vi "Monitors_EPR_v02.vi"(0 "IIR filter specifications":T1={"Topology"=enum."Butterworth", "Type"=enum."Lowpass", "Order"=1, "Lower Fc"=100.0, "Upper Fc"=200.0, "PB Ripple"=1.0, "SB Attenuation"=60.0} {"PB Ripple" format="%0.2f"; "SB Attenuation" format="%0.2f"; "Lower Fc" format="%0.2p"; "Upper Fc" format="%0.2p"}, 3 "Wait(mSec)":u32 caption="Count(mSec)", 5 "reset SN":bool, 7 "mode 2 polarity(T=+ve)":bool, 9 "Shot noise start":bool, 11 "wfm":waveform(dbl)[](array[waveform]), 12 "mode 3 polarity(T=+ve)":bool) -> (4 "Var(x1-x2/sqrt(2)-x3/sqrt(2))":dbl, 6 "Var(x2-x1/sqrt(2)-x3/sqrt(2))":dbl, 8 "Var(x3-x1/sqrt(2)-x2/sqrt(2))":dbl)   [LabVIEW 2013]
uses:
  <vilib>/Analysis/5stat.llb/RMS (DBL).vi
  shotnoise.vi
  <vilib>/measure/maspectr.llb/FFT Spectrum (Mag-Phase) for N Chan.vi
  <vilib>/measure/matone.llb/Extract Single Tone Information N Chan.vi
  <vilib>/measure/macond.llb/IIR Filter for N Chan.vi
  <vilib>/measure/NI_MAPro.lvlib
  <vilib>/Analysis/NI_AALPro.lvlib
panel:
  out "Waveform Graph 2":cluster{"f0":dbl, "df":dbl, "magnitude":dbl[]}[](graph)
  out "detected frequencies":dbl[](array[numeric]) format="%.2p"
  out "ch12":dbl
  out "ch02":dbl
  out "ch01":dbl
  out "Waveform Graph":waveform(dbl)[](graph)
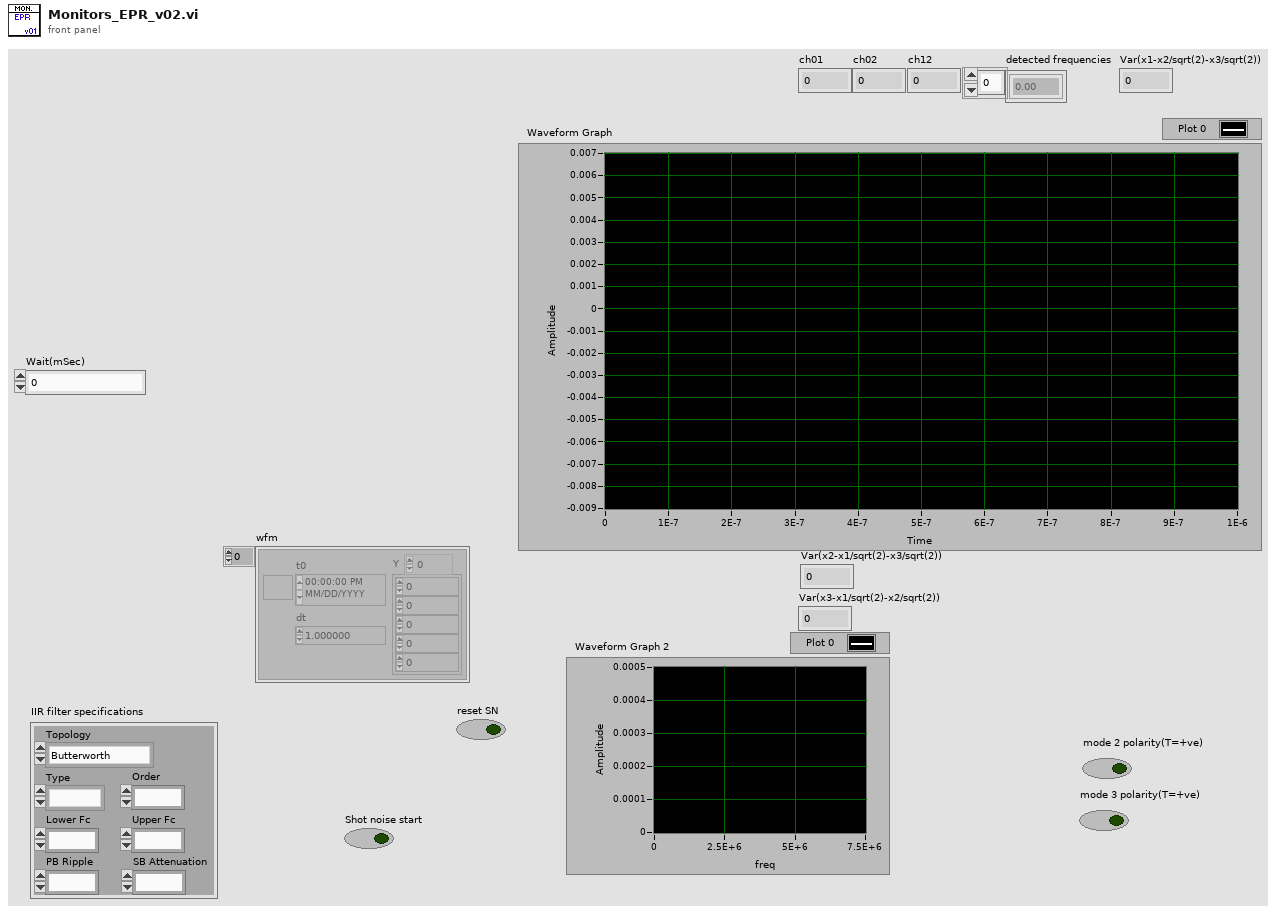
[diagram p1: front panel]
types:
  T1 = cluster{"Topology":enum16{"Off", "Butterworth", "Chebyshev", "Inverse Chebyshev", "Elliptic", "Bessel"}, "Type":enum16{"Lowpass", "Highpass", "Bandpass", "Bandstop"}, "Order":i32, "Lower Fc":dbl, "Upper Fc":dbl, "PB Ripple":dbl, "SB Attenuation":dbl}
  T2 = cluster{"approx freq. (optional)":dbl, "search (+/- % of Fsampl.)":dbl}
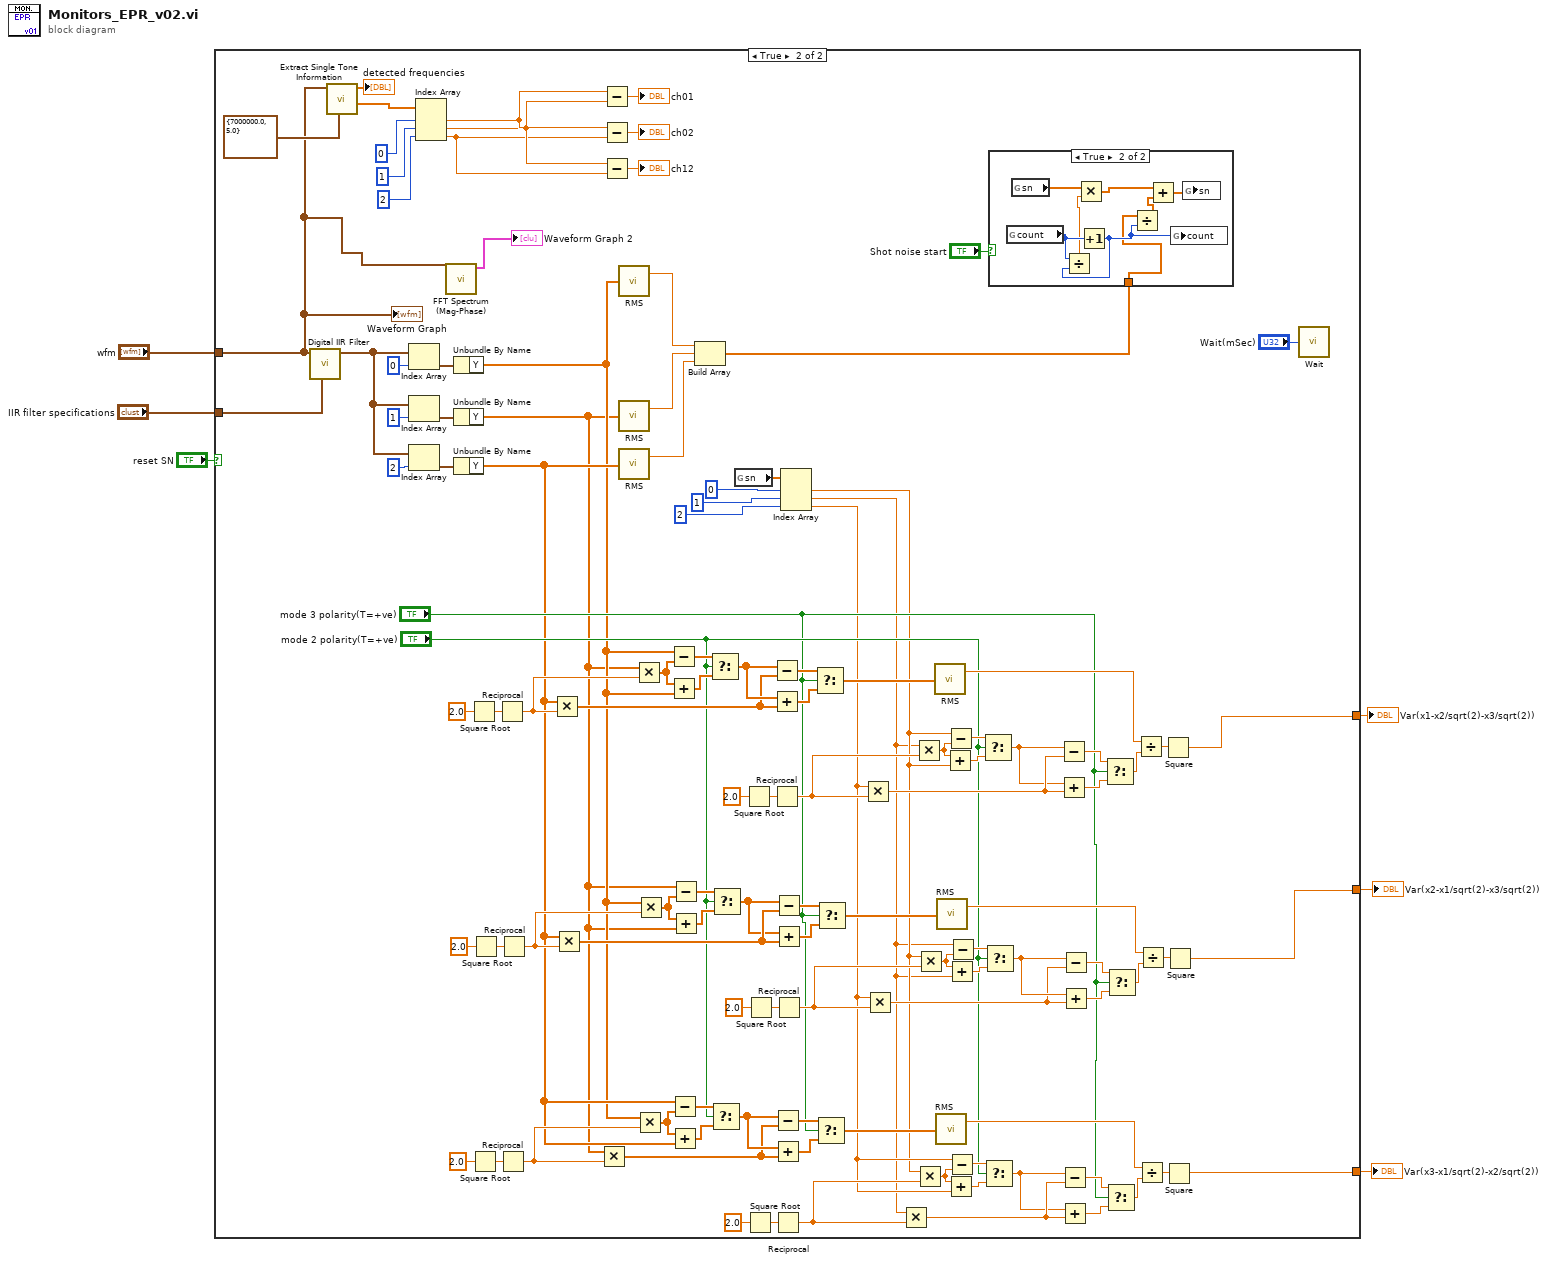
[diagram p0: block diagram]
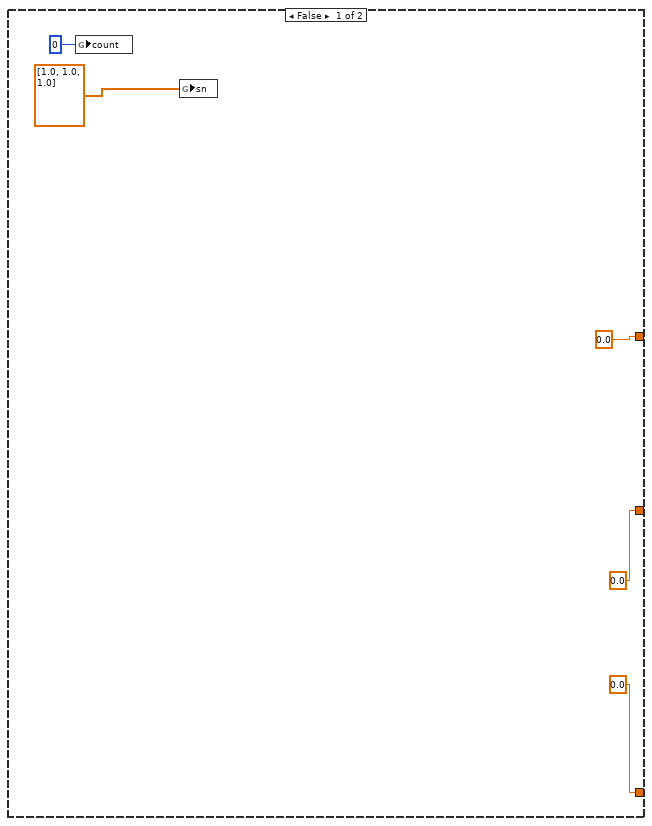
[diagram p2: hidden frame]
diagram:
  n1 = case shown="True" "reset SN" {
    tunnel: "IIR filter specifications" -> [_ w126]
    tunnel: "wfm" -> [_ w95]
    tunnel: [0.0 w89] -> w3
    tunnel: [0.0 w45] -> w2
    tunnel: [0.0 w12] -> w1
    frame False {
      n2 = global write "shotnoise.vi" "count"(i64 0 ("count")) -> ()
      n3 = global write "shotnoise.vi" "sn"(dbl[] [1.0, 1.0, 1.0] ("sn")) -> ()
    }
    frame True {
      n4 = call-poly <vilib>:"Digital IIR Filter.vi"("IIR filter specifications"=w126, "signal(s) in"=w95) -> ("signal(s) out"=w114:waveform(dbl)[])  [unwired: 4 in, 5 out]
      n5 = call-poly <vilib>:"Extract Single Tone Information.vi"("advanced search"=T2 {"approx freq. (optional)"=7000000.0, "search (+/- % of Fsampl.)"=5.0}, "time signals in"=w95) -> ("detected phases (deg)"=w105:dbl[], "detected frequencies"=→"detected frequencies":dbl[])  [unwired: 4 in, 4 out]
      n6 = Index Array(array=w114, index=0) -> (element=w118:waveform(dbl))
      n7 = Index Array(array=w114, index=1) -> (element=w121:waveform(dbl))
      n8 = Index Array(array=w114, index=2) -> (element=w113:waveform(dbl))
      n9 = Index Array(array=w105, index #1=0 ("index"), index #2=1 ("index"), index #3=2 ("index")) -> (element #1=w104:dbl, element #2=w103:dbl, element #3=w102:dbl)
      n10 = call-poly <vilib>:"FFT Spectrum (Mag-Phase).vi"("time signals"=w95) -> ("magnitudes"=→"Waveform Graph 2":cluster{"f0":dbl, "df":dbl, "magnitude":dbl[]}[])  [unwired: 6 in, 4 out]
      n11 = Unbundle By Name(w118) -> ("Y"=w16:dbl[])
      n12 = Unbundle By Name(w121) -> ("Y"=w13:dbl[])
      n13 = Unbundle By Name(w113) -> ("Y"=w18:dbl[])
      n14 = Square Root(x=2.0) -> (sqrt(x)=w93:dbl)
      n15 = Square Root(x=2.0) -> (sqrt(x)=w43:dbl)
      n16 = Square Root(x=2.0) -> (sqrt(x)=w47:dbl)
      n17 = Reciprocal(x=w93) -> (1/x=w87:dbl)
      n18 = Reciprocal(x=w43) -> (1/x=w38:dbl)
      n19 = Reciprocal(x=w47) -> (1/x=w52:dbl)
      n20 = Multiply(x=w18, y=w87) -> (x*y=w81:dbl[])
      n21 = Multiply(x=w18, y=w52) -> (x*y=w58:dbl[])
      n22 = Multiply(x=w13, y=w38) -> (x*y=w32:dbl[])
      n23 = Subtract(x=w104, y=w103) -> (x-y=→"ch01":dbl)
      n24 = Subtract(x=w104, y=w102) -> (x-y=→"ch02":dbl)
      n25 = Subtract(x=w103, y=w102) -> (x-y=→"ch12":dbl)
      n26 = call-poly <vilib>:"RMS.vi"("X"=w16) -> ("rms value"=w124:dbl)  [unwired: 1 out]
      n27 = call-poly <vilib>:"RMS.vi"("X"=w13) -> ("rms value"=w125:dbl)  [unwired: 1 out]
      n28 = call-poly <vilib>:"RMS.vi"("X"=w18) -> ("rms value"=w110:dbl)  [unwired: 1 out]
      n29 = Multiply(x=w13, y=w87) -> (x*y=w85:dbl[])
      n30 = Multiply(x=w16, y=w38) -> (x*y=w36:dbl[])
      n31 = Multiply(x=w16, y=w52) -> (x*y=w54:dbl[])
      n32 = Subtract(x=w16, y=w85) -> (x-y=w84:dbl[])
      n33 = Add(x=w85, y=w16) -> (x+y=w83:dbl[])
      n34 = Subtract(x=w18, y=w36) -> (x-y=w35:dbl[])
      n35 = Add(x=w36, y=w18) -> (x+y=w34:dbl[])
      n36 = Subtract(x=w13, y=w54) -> (x-y=w55:dbl[])
      n37 = Add(x=w54, y=w13) -> (x+y=w56:dbl[])
      n38 = Build Array(w124, w125, w110) -> (w123:dbl[])
      n39 = Select(t=w84, s="mode 2 polarity(T=+ve)", f=w83) -> (s? t:f=w82:dbl[])
      n40 = Select(t=w35, s="mode 2 polarity(T=+ve)", f=w34) -> (s? t:f=w33:dbl[])
      n41 = Select(t=w55, s="mode 2 polarity(T=+ve)", f=w56) -> (s? t:f=w57:dbl[])
      n42 = global read "shotnoise.vi" "sn"() -> (w120:dbl[])
      n43 = Square Root(x=2.0) -> (sqrt(x)=w92:dbl)
      n44 = Square Root(x=2.0) -> (sqrt(x)=w42:dbl)
      n45 = Square Root(x=2.0) -> (sqrt(x)=w48:dbl)
      n46 = Subtract(x=w82, y=w81) -> (x-y=w79:dbl[])
      n47 = Add(x=w82, y=w81) -> (x+y=w80:dbl[])
      n48 = Reciprocal(x=w92) -> (1/x=w86:dbl)
      n49 = Subtract(x=w33, y=w32) -> (x-y=w30:dbl[])
      n50 = Add(x=w33, y=w32) -> (x+y=w31:dbl[])
      n51 = Reciprocal(x=w42) -> (1/x=w37:dbl)
      n52 = Subtract(x=w57, y=w58) -> (x-y=w60:dbl[])
      n53 = Add(x=w57, y=w58) -> (x+y=w59:dbl[])
      n54 = Reciprocal(x=w48) -> (1/x=w53:dbl)
      n55 = Index Array(array=w120, index #1=0 ("index"), index #2=1 ("index"), index #3=2 ("index")) -> (element #1=w15:dbl, element #2=w14:dbl, element #3=w17:dbl)
      n56 = Select(t=w79, s="mode 3 polarity(T=+ve)", f=w80) -> (s? t:f=w78:dbl[])
      n57 = Select(t=w30, s="mode 3 polarity(T=+ve)", f=w31) -> (s? t:f=w29:dbl[])
      n58 = Select(t=w60, s="mode 3 polarity(T=+ve)", f=w59) -> (s? t:f=w61:dbl[])
      n59 = Multiply(x=w17, y=w86) -> (x*y=w74:dbl)
      n60 = Multiply(x=w17, y=w53) -> (x*y=w65:dbl)
      n61 = Multiply(x=w14, y=w37) -> (x*y=w25:dbl)
      n62 = Multiply(x=w14, y=w86) -> (x*y=w77:dbl)
      n63 = Multiply(x=w15, y=w37) -> (x*y=w28:dbl)
      n64 = Multiply(x=w15, y=w53) -> (x*y=w62:dbl)
      n65 = call-poly <vilib>:"RMS.vi"("X"=w78) -> ("rms value"=w88:dbl)  [unwired: 1 out]
      n66 = call-poly <vilib>:"RMS.vi"("X"=w29) -> ("rms value"=w39:dbl)  [unwired: 1 out]
      n67 = call-poly <vilib>:"RMS.vi"("X"=w61) -> ("rms value"=w51:dbl)  [unwired: 1 out]
      n68 = Add(x=w77, y=w15) -> (x+y=w75:dbl)
      n69 = Subtract(x=w15, y=w77) -> (x-y=w76:dbl)
      n70 = Add(x=w28, y=w17) -> (x+y=w26:dbl)
      n71 = Add(x=w62, y=w14) -> (x+y=w64:dbl)
      n72 = Subtract(x=w17, y=w28) -> (x-y=w27:dbl)
      n73 = Subtract(x=w14, y=w62) -> (x-y=w63:dbl)
      n74 = Select(t=w76, s="mode 2 polarity(T=+ve)", f=w75) -> (s? t:f=w73:dbl)
      n75 = Select(t=w27, s="mode 2 polarity(T=+ve)", f=w26) -> (s? t:f=w24:dbl)
      n76 = Select(t=w63, s="mode 2 polarity(T=+ve)", f=w64) -> (s? t:f=w66:dbl)
      n77 = case shown="True" "Shot noise start" {
        tunnel: w123 -> [_ w128]
        frame False {
        }
        frame True {
          n78 = global read "shotnoise.vi" "count"() -> (w133:i64)
          n79 = global read "shotnoise.vi" "sn"() -> (w132:dbl[])
          n80 = Increment(x=w133) -> (x+1=w129:i64)
          n81 = Divide(x=w133, y=w129) -> (x/y=w131:dbl)
          n82 = Multiply(x=w132, y=w131) -> (x*y=w130:dbl[])
          n83 = Divide(x=w128, y=w129) -> (x/y=w127:dbl[])
          n84 = Add(x=w130, y=w127) -> (x+y=w134:dbl[])
          n85 = global write "shotnoise.vi" "count"(w129) -> ()
          n86 = global write "shotnoise.vi" "sn"(w134) -> ()
        }
      }
      n87 = Subtract(x=w73, y=w74) -> (x-y=w71:dbl)
      n88 = Add(x=w73, y=w74) -> (x+y=w72:dbl)
      n89 = Subtract(x=w24, y=w25) -> (x-y=w22:dbl)
      n90 = Add(x=w24, y=w25) -> (x+y=w23:dbl)
      n91 = Subtract(x=w66, y=w65) -> (x-y=w68:dbl)
      n92 = Add(x=w66, y=w65) -> (x+y=w67:dbl)
      n93 = Select(t=w71, s="mode 3 polarity(T=+ve)", f=w72) -> (s? t:f=w70:dbl)
      n94 = Select(t=w22, s="mode 3 polarity(T=+ve)", f=w23) -> (s? t:f=w21:dbl)
      n95 = Select(t=w68, s="mode 3 polarity(T=+ve)", f=w67) -> (s? t:f=w69:dbl)
      n96 = Divide(x=w88, y=w70) -> (x/y=w90:dbl)
      n97 = Divide(x=w39, y=w21) -> (x/y=w40:dbl)
      n98 = Divide(x=w51, y=w69) -> (x/y=w50:dbl)
      n99 = Square(x=w90) -> (x^2=w89:dbl)
      n100 = Square(x=w40) -> (x^2=w12:dbl)
      n101 = Square(x=w50) -> (x^2=w45:dbl)
      n102 = call "Wait"("Count(mSec)"="Wait(mSec)") -> ()  [unwired: 1 out]
      "Waveform Graph" <- w95
    }
  }
  "Var(x1-x2/sqrt(2)-x3/sqrt(2))" <- w3
  "Var(x2-x1/sqrt(2)-x3/sqrt(2))" <- w2
  "Var(x3-x1/sqrt(2)-x2/sqrt(2))" <- w1
